vi "u64 to cpx number.vi"(11 "Numeric":u64) -> (1 "x + iy":cdb)   [LabVIEW 2020]
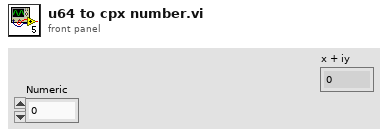
[diagram p1: front panel]
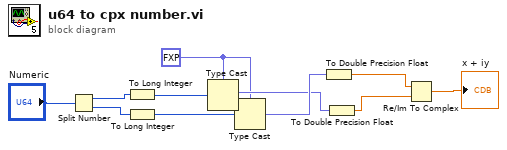
[diagram p0: block diagram]
diagram:
  w7 = fxp<+/-,32,11> 0.0 ("Number of Elements")
  n1 = Split Number(x="Numeric") -> (hi(x)=w4:u32, lo(x)=w5:u32)
  n2 = To Long Integer(number=w4) -> (32bit integer=w6:i32)
  n3 = To Long Integer(number=w5) -> (32bit integer=w10:i32)
  n4 = Type Cast(type=w7, x=w6) -> (*(type *) &x=w8:fxp<+/-,32,11>)
  n5 = Type Cast(type=w7, x=w10) -> (*(type *) &x=w11:fxp<+/-,32,11>)
  n6 = To Double Precision Float(number=w11) -> (double precision float=w3:dbl)
  n7 = To Double Precision Float(number=w8) -> (double precision float=w2:dbl)
  n8 = Re/Im To Complex(1:w2, 2:w3) -> (0:→"x + iy":cdb)
